vi "Save Copy of Template Library.vi"(8 "error in":errorcluster, 9 "plugin name":string, 10 "template library path":path, 11 "project path":path) -> (0 "error out":errorcluster, 3 "plugin library path":path)   [LabVIEW 2021, in "InstrumentStudio Plug-In Editor.lvlib"]
uses:
  InstrumentStudio Plug-In Editor.lvlib
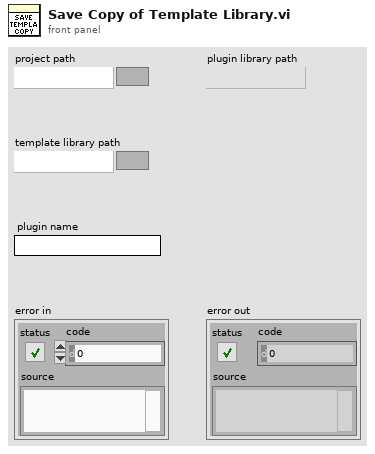
[diagram p1: front panel]
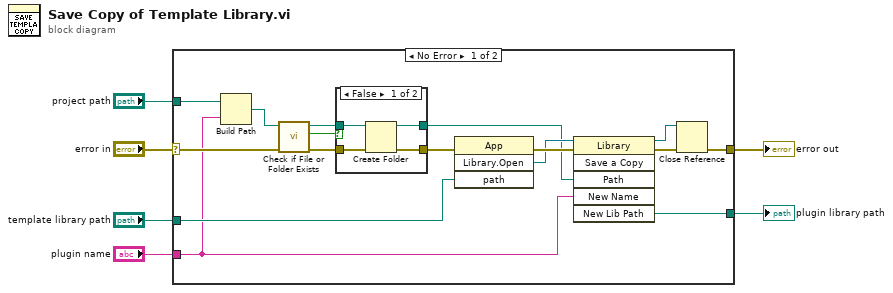
[diagram p0: block diagram]
diagram:
  n1 = case shown="No Error" "error in" {
    selector: "error in" -> [w13 w29]
    tunnel: "template library path" -> [w22 _]
    tunnel: [w20 w29] -> w5
    tunnel: "project path" -> [w11 _]
    tunnel: "plugin name" -> [w10 _]
    tunnel: [w9 _] -> w1
    frame No Error {
      n2 = Build Path(base path=w11, name or relative path=w10) -> (appended path=w12:path)
      n3 = call <vilib>:"Check if File or Folder Exists.vi"("error in (no error)"=w13, "path"=w12) -> ("error out"=w14:errorcluster, "file or folder exists?"=w16:bool, "dup path"=w15:path)  [unwired: 7 in]
      n4 = case shown="False" w16 {
        tunnel: w14 -> [w26 w27]
        tunnel: w15 -> [w25 w28]
        tunnel: [w24 w28] -> w7
        tunnel: [w23 w27] -> w21
        frame False {
          n5 = Create Folder(path (use dialog)=w25, error in=w26) -> (created path=w24:path, error out=w23:errorcluster)  [unwired: 1 in, 1 out]
        }
        frame True {
        }
      }
      n6 = invoke class="App" method="Library.Open"(error in=w21, "path"=w22) -> (error out=w18:errorcluster, "Open Library"=w8:refnum<vi>)  [unwired: 2 in, 2 out]
      n7 = invoke class="Library" method="Save a Copy"(reference=w8, error in=w18, "Path"=w7, "New Name"=w10) -> (reference out=w17:refnum<vi>, error out=w19:errorcluster, "New Lib Path"=w9:path)  [unwired: 2 in, 3 out]
      n8 = Close Reference(reference=w17, error in (no error)=w19) -> (error out=w20:errorcluster)
    }
    frame Error {
    }
  }
  "plugin library path" <- w1
  "error out" <- w5
